vi "Find TestReport Directory.vi"(8 "error in (no error)":errorcluster) -> (0 "error out":errorcluster, 1 "Exists?":bool, 3 "Test Report Directory":path)   [LabVIEW 2015]
doc: "Find the parent directory for the example. TestStand needs this information to properly call VIs in the application.\n____\nDelacor QMH Thermal Chamber Examples 4.0.0.21\nCopyright (c) 2018, Delacor"
uses:
  <vilib>/Utility/error.llb/Error Cluster From Error Code.vi
  <vilib>/ErrorRing/Error Ring.xnode
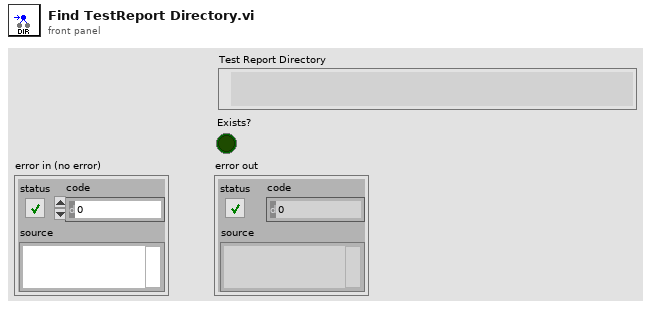
[diagram p1: front panel]
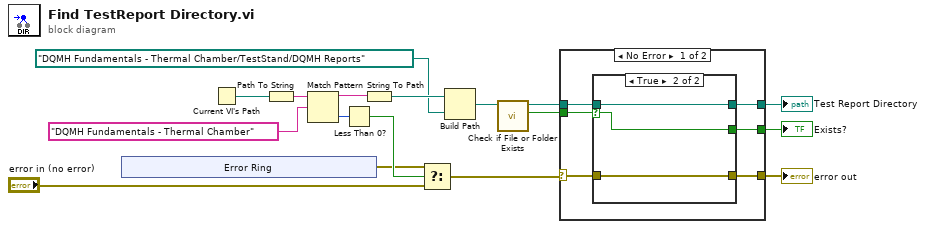
[diagram p0: block diagram]
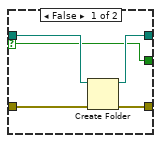
[diagram p2: hidden frame]
diagram:
  n1 = xnode "Error Ring"() -> ("error out"=w11:errorcluster)
  n2 = Current VI's Path() -> (path=w17:path)
  n3 = Path To String(path=w17) -> (string=w16:string)
  n4 = Match Pattern(string=w16, regular expression="DQMH Fundamentals - Thermal Chamber") -> (before substring=w15:string, offset past match=w13:i32)  [unwired: 1 in, 2 out]
  n5 = Less Than 0?(x=w13) -> (x < 0?=w12:bool)
  n6 = String To Path(string=w15) -> (path=w14:path)
  n7 = Select(t=w11, s=w12, f="error in (no error)") -> (s? t:f=w3:errorcluster)
  n8 = Build Path(base path=w14, name or relative path=path "DQMH Fundamentals - Thermal Chamber/TestStand/DQMH Reports") -> (appended path=w9:path)
  n9 = call <vilib>:"Check if File or Folder Exists.vi"("path"=w9) -> ("file or folder exists?"=w8:bool, "dup path"=w7:path)  [unwired: 8 in, 1 out]
  n10 = case shown="No Error" w3 {
    selector: w3 -> [w20 w32]
    tunnel: w8 -> [w23 _]
    tunnel: w7 -> [w22 _]
    tunnel: [w21 _] -> w6
    tunnel: [w19 w32] -> w2
    tunnel: [w18 _] -> w1
    frame No Error {
      n11 = case shown="True" w23 {
        selector: w23 -> [w24 w29]
        tunnel: w22 -> [w26 w31]
        tunnel: [w25 w31] -> w21
        tunnel: w20 -> [w28 w30]
        tunnel: [w27 w30] -> w19
        tunnel: [w24 w29] -> w18
        frame False {
          n12 = Create Folder(path (use dialog)=w26, error in=w28) -> (created path=w25:path, error out=w27:errorcluster)  [unwired: 1 in, 1 out]
        }
        frame True {
        }
      }
    }
    frame Error {
    }
  }
  "error out" <- w2
  "Exists?" <- w1
  "Test Report Directory" <- w6
